vi "CANopencRIOSDODemo.vi"() -> ()   [LabVIEW 2016]
doc: "Read SDO Information.\nThis example is written for a WAGO 750-307 device."
uses:
  <vilib>/FPGAPlugInAG/cRIO-9033/niLvFpga_Close_cRIO-9033.vi
  <vilib>/rvi/interface/nirviCloseFPGA/nirviCloseFPGA.xnode
  FPGA Bitfiles/EV-MCU_FPGATarget_CANEngine(FPGA)b_eM8Xz3qYJVA.lvbitx
  CAN_Engine(FPGA)_basic.vi
panel:
  out "Data":u8[](array[numeric])
  in  "Sub Index":u8 format="%.0x"
  in  "Index":u16=4104 format="%.0x"
  out "Data (ASCII)":string
  out "error out":errorcluster
  # "Project uses 500 Kbaud\nand node ID 1"
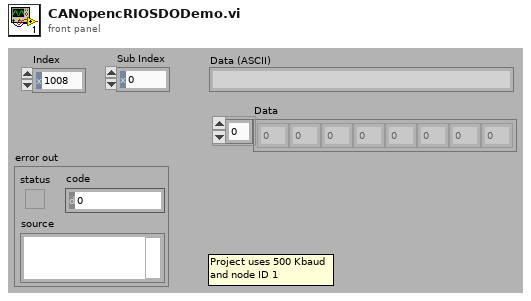
[diagram p1: front panel]
types:
  T1 = enum16{"start remote node", "stop remote node", "reset node", "reset communication", "enter preoperational"}
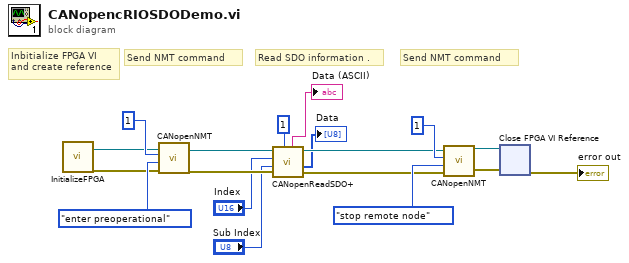
[diagram p0: block diagram]
diagram:
  # "Read SDO information ."
  # "Send NMT command"
  # "Send NMT command"
  # "Inbitialize FPGA VI \nand create reference"
  n1 = call "InitializeFPGA.vi"() -> ("error out"=w15:errorcluster, "FPGA VI Reference Out"=w14:refnum<k20>)  [unwired: 2 in]
  n2 = call "CANopenNMT.vi"("error in"=w15, "Mode"=T1."enter preoperational", "Node ID"=u8 1, "FPGA VI Reference In"=w14) -> ("error out"=w7:errorcluster, "FPGA VI Reference Out"=w9:refnum<k20>)
  n3 = call "CANopenReadSDO+.vi"("Node ID"=u32 1, "error in"=w7, "Sub Index"="Sub Index", "Index"="Index", "FPGA VI Reference In"=w9) -> ("error out"=w6:errorcluster, "Data"=→"Data":u8[], "FPGA VI Reference Out"=w8:refnum<k20>, "Data (ASCII)"=→"Data (ASCII)":string)  [unwired: 1 in]
  n4 = call "CANopenNMT.vi"("error in"=w6, "Mode"=T1."stop remote node", "Node ID"=u8 1, "FPGA VI Reference In"=w8) -> ("error out"=w12:errorcluster, "FPGA VI Reference Out"=w11:refnum<k20>)
  n5 = xnode "Close FPGA VI Reference"("FPGA VI Reference In"=w11, "error in"=w12) -> ("error out"=→"error out":errorcluster)
